vi "Test_Accel.vi"() -> ()   [LabVIEW 2017]
uses:
  <vilib>/Analysis/NI_AALPro.lvlib
panel:
  out "Integral X":dbl[](array[numeric])
  out "Waveform Chart 3":dbl[](graph)
  out "Waveform Chart 2":dbl[](graph)
  in  "stop":bool
  in  "Samples qty":i32
  in  "Period (ms)":u32=10
  in  "COM Port":refnum<visa-resource-name>="COM1"
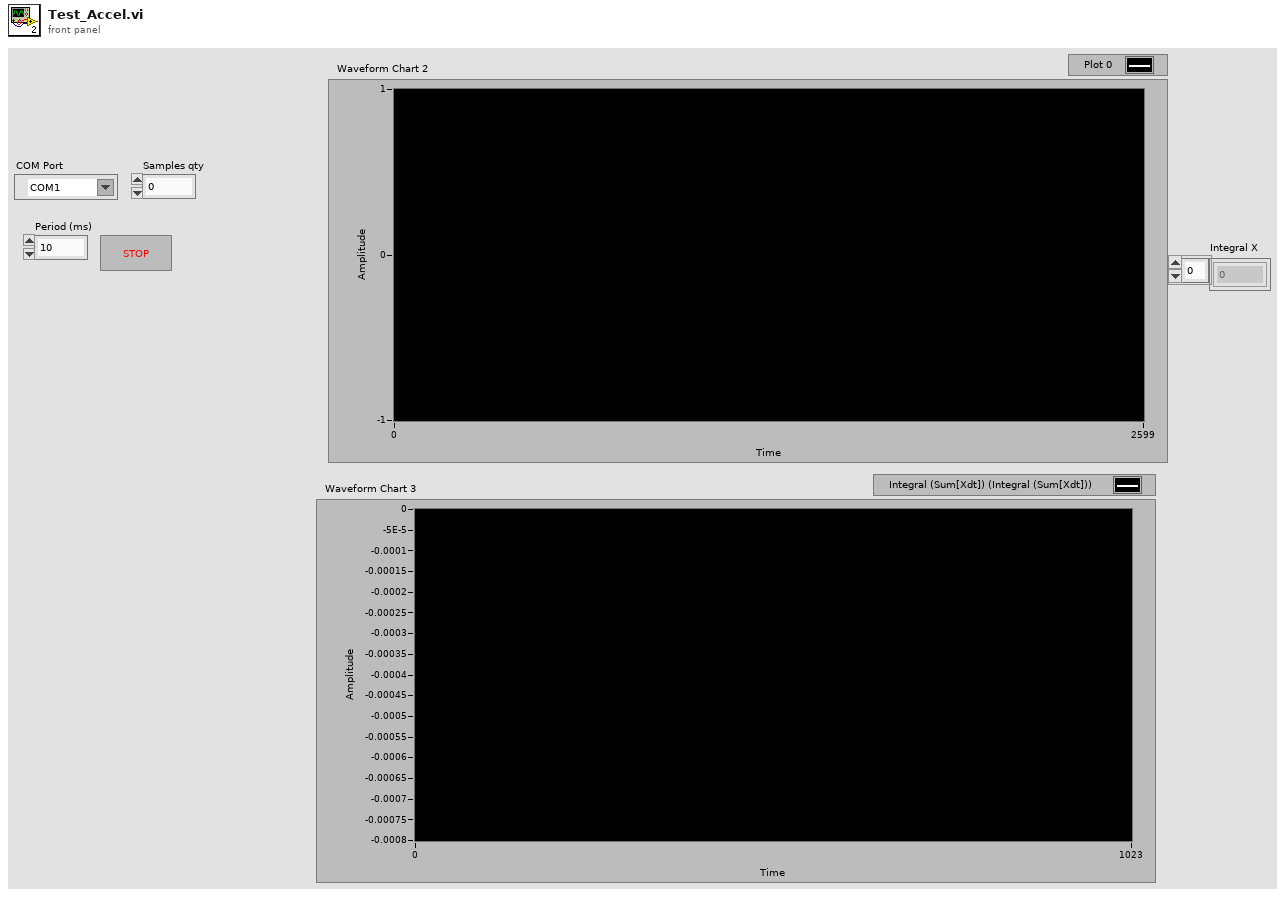
[diagram p1: front panel]
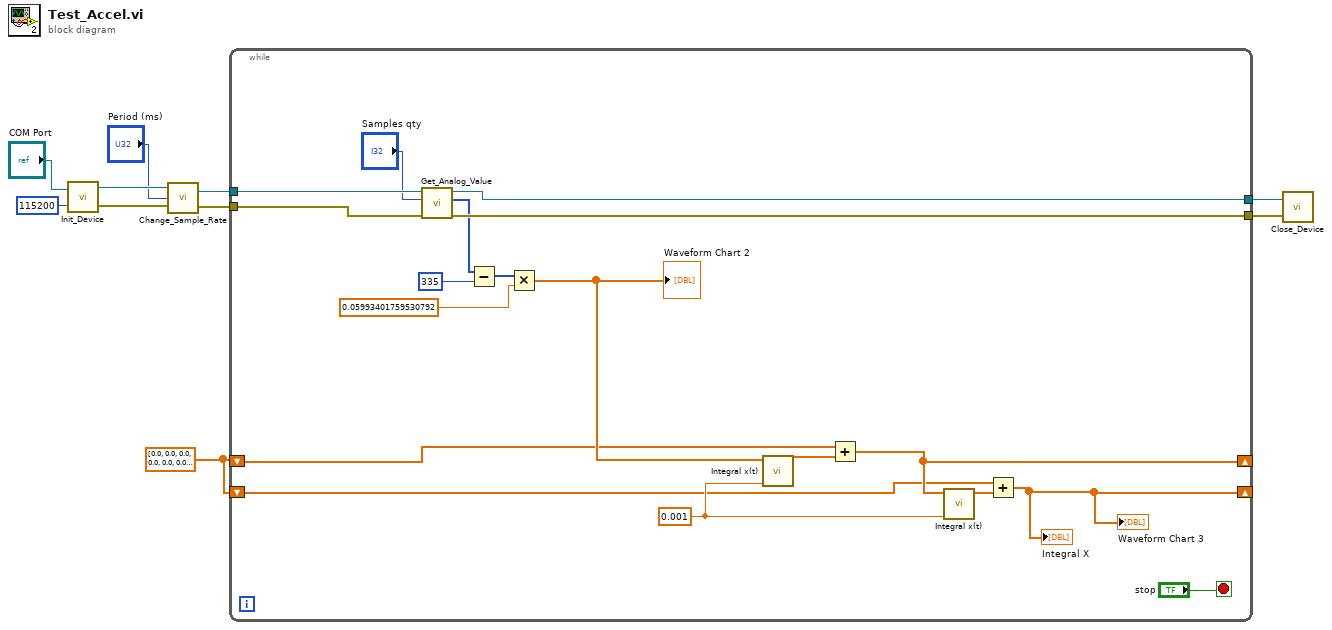
[diagram p0: block diagram]
diagram:
  w1 = dbl[] [0.0, 0.0, 0.0, 0.0, 0.0, 0.0, 0.0, 0.0, 0.0, 0.0, 0.0, 0.0, 0.0, 0.0, 0.0, 0.0, 0.0, 0.0, 0.0, 0.0, 0.0, 0.0, 0.0, 0.0, 0.0, 0.0, 0.0, 0.0, 0.0, 0.0, 0.0, 0.0, 0.0, 0.0, 0.0, 0.0, 0.0, 0.0, 0.0, 0.0, 0.0, 0.0, 0.0, 0.0, 0.0, 0.0, 0.0, 0.0, 0.0, 0.0, 0.0, 0.0, 0.0, 0.0, 0.0, 0.0, 0.0, 0.0, 0.0, 0.0, 0.0, 0.0, 0.0, 0.0, 0.0, 0.0, 0.0, 0.0, 0.0, 0.0, 0.0, 0.0, 0.0, 0.0, 0.0, 0.0, 0.0, 0.0, 0.0, 0.0, 0.0, 0.0, 0.0, 0.0, 0.0, 0.0, 0.0, 0.0, 0.0, 0.0, 0.0, 0.0, 0.0, 0.0, 0.0, 0.0, 0.0, 0.0, 0.0, 0.0]
  n1 = call "Init_Device.vi"("Baud Rate"=u32 115200, "COM Port"="COM Port") -> ("error out"=w7:errorcluster, "Device Session"=w8:refnum<visa-resource-name>)
  n2 = call "Change_Sample_Rate.vi"("error in"=w7, "Period (ms)"="Period (ms)", "Device Session In"=w8) -> ("error out"=w6:errorcluster, "Device Session Out"=w5:refnum<visa-resource-name>)
  n3 = while {
    tunnel: w6 -> [w28]
    tunnel: w5 -> [w27]
    tunnel: [w24] -> w3
    tunnel: [w23] -> w2
    shift-right: [w12] -> _
    shift-left: w1 -> [w11]
    shift-right: [w15] -> _
    shift-left: w1 -> [w14]
    stop <- "stop" stop-if-true
    w20 = 0.001 ("dt")
    n4 = call "Get_Analog_Value.vi"("error in"=w28, "Samples qty"="Samples qty", "Device Session In"=w27) -> ("error out"=w24:errorcluster, "Output values"=w21:i32[], "Device Session Out"=w23:refnum<visa-resource-name>)  [unwired: 5 in]
    n5 = Subtract(x=w21, y=335) -> (x-y=w19:i32[])
    n6 = Multiply(x=w19, y=0.05993401759530792 ("dt")) -> (x*y=w17:dbl[])
    "Waveform Chart 2" <- w17
    n7 = call <vilib>:"Integral x(t).vi"("dt"=w20, "X"=w17) -> ("Integral X"=w16:dbl[])  [unwired: 8 in, 1 out]
    n8 = Add(x=w14, y=w16) -> (x+y=w15:dbl[])
    n9 = call <vilib>:"Integral x(t).vi"("dt"=w20, "X"=w15) -> ("Integral X"=w13:dbl[])  [unwired: 8 in, 1 out]
    n10 = Add(x=w11, y=w13) -> (x+y=w12:dbl[])
    "Waveform Chart 3" <- w12
    "Integral X" <- w12
  }
  n11 = call "Close_Device.vi"("error in"=w3, "Device Session"=w2) -> ()  [unwired: 1 in, 1 out]
